vi "FTW-Connector-Construct.vi"(5 "Remote Inbox Address":string, 7 "Receive Message Size Limit":i32=1000000 format="%_4pbytes", 11 "error in":errorcluster) -> (4 "FTW Actor Connector":T1, 15 "error out":errorcluster)   [LabVIEW 2015]
doc: "Performs a \"cold call\" to connect to a running Actor Instance at the given Instance Inbox Address. Normally, this method is wrapped by a \"Construct\" method in each specific Actor Connector subclass."
uses:
  core/type/FTW-Type-Actor-Connector.ctl
panel:
  # "Inputs"
  # "Outputs"
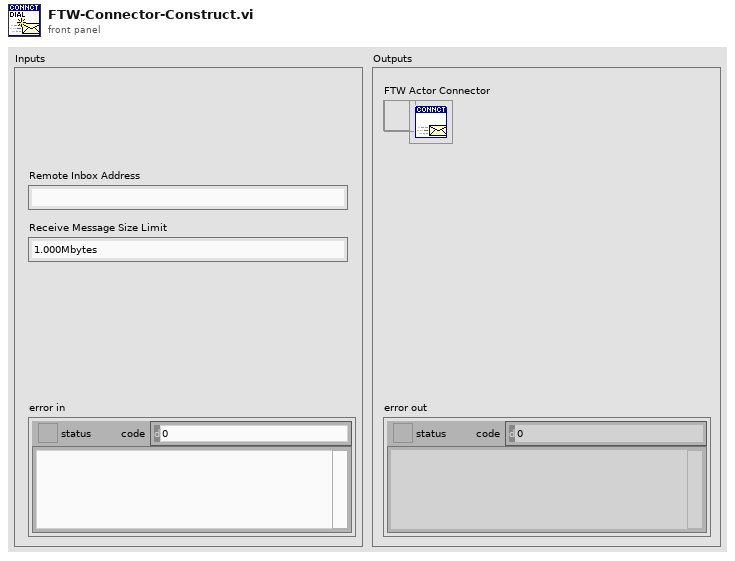
[diagram p1: front panel]
types:
  T1 = typedef "FTW-Type-Actor-Connector.ctl" = refnum<data-value>
  T2 = cluster{"FTW-CodeGen-Type":enum16{"FTW-Actor-Connector"}, "Socket":i64}
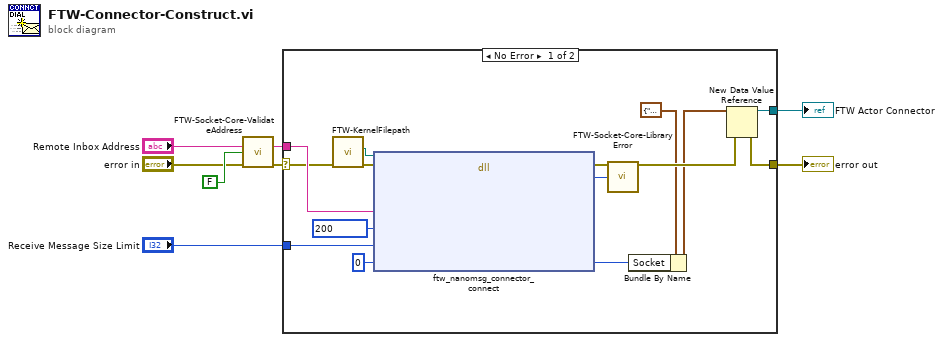
[diagram p0: block diagram]
diagram:
  n1 = call "FTW-Socket-Core-ValidateAddress.vi"("Address"="Remote Inbox Address", "Allow wildcard replacement?"=FALSE, "error in"="error in") -> ("Sanitized Address"=w3:string, "error out"=w4:errorcluster)  [unwired: 10 in, 1 out]
  n2 = case shown="No Error" w4 {
    selector: w4 -> [w13 w24]
    tunnel: [w22 w24] -> w8
    tunnel: w3 -> [w19 _]
    tunnel: [w21 _] -> w7
    tunnel: "Receive Message Size Limit" -> [w16 _]
    frame No Error {
      n3 = call "FTW-KernelFilepath.vi"("error in"=w13) -> ("error out"=w12:errorcluster, "Library Filepath"=w11:path)  [unwired: 8 in, 1 out]
      n4 = dll-call lib="?" fn="ftw_nanomsg_connector_connect"(path in=w11, error in=w12, "Remote Address"=w19, "Linger (msec)"=200 ("Linger"), "Max Recv Size (bytes)"=w16, "Socket Handle"=i64 0) -> (error out=w20:errorcluster, "Return Value"=w17:i64, "Socket Handle"=w14:i64)  [unwired: 6 in, 1 out]
      n5 = call "FTW-Socket-Core-LibraryError.vi"("error in"=w20, "Return Value"=w17) -> ("error out"=w23:errorcluster)  [unwired: 13 in]
      n6 = Bundle By Name(cluster=T2 {"FTW-CodeGen-Type"=enum."FTW-Actor-Connector", "Socket"=0}, "Socket"=w14) -> (w15:T2)
      n7 = New Data Value Reference(data value=w15, error in=w23) -> (data value reference=w21:refnum<data-value>, error out=w22:errorcluster)
    }
    frame Error {
    }
  }
  "error out" <- w8
  "FTW Actor Connector" <- w7
